vi "midiInOpen.vi"(7 "Event Filter":u8[](array[numeric])=[128, 144, 176] format="%.0x", 8 "error in":errorcluster, 9 "MidiDataEvents":refnum<user-event>, 10 "MIDI Device ID":u32, 11 "midi in":refnum<class "midi.lvclass">) -> (0 "error out":errorcluster, 3 "midi out":refnum<class "midi.lvclass">)   [LabVIEW 2020, in "midi.lvclass"]
doc: "The midiInOpen function opens a specified MIDI input device."
uses:
  midi.lvclass
  midi.lvclass/midi.ctl
  cpp-src/MIDIInToLabVIEWWrapper/x64/Release/MIDIInToLabVIEWWrapper.dll
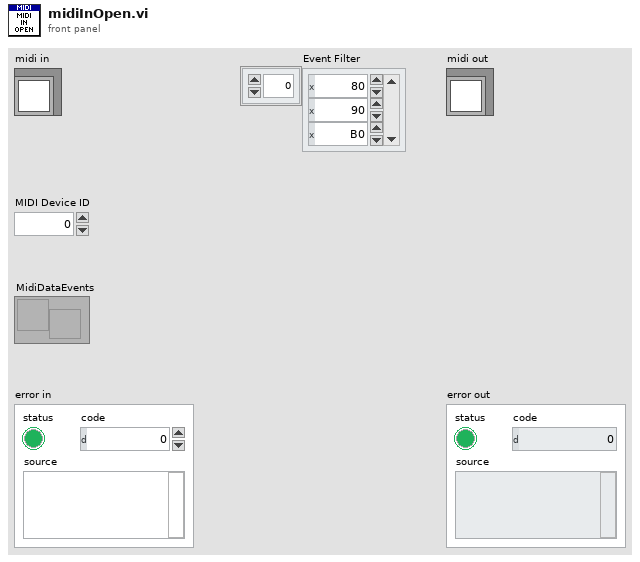
[diagram p1: front panel]
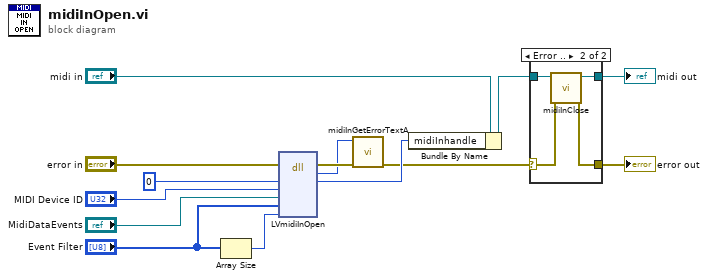
[diagram p0: block diagram]
diagram:
  n1 = Array Size(array="Event Filter") -> (size(s)=w2:i32)
  n2 = dll-call lib="C:/code/LabVIEW-MIDI/cpp-src/MIDIInToLabVIEWWrapper/x64/Release/MIDIInToLabVIEWWrapper.dll" fn="LVmidiInOpen"(error in="error in", "phMidiIn"=u64 0 ("hMidiIn"), "uDeviceID"="MIDI Device ID", "pUserEventRef"="MidiDataEvents", "filterArray"="Event Filter", "arraySize"=w2) -> (error out=w8:errorcluster, "error"=w7:i32, "phMidiIn"=w6:u64)  [unwired: 6 in, 1 out]
  n3 = call "midiInGetErrorTextA.vi"("error in"=w8, "Error Code"=w7) -> ("error out"=w5:errorcluster)  [unwired: 9 in]
  n4 = Bundle By Name(cluster="midi in", "midiInhandle"=w6) -> (w13:refnum<class "midi.lvclass">)
  n5 = case shown="Error .." w5 {
    selector: w5 -> [w15 w17]
    tunnel: w13 -> [w16 w20]
    tunnel: [w16 w19] -> w12
    tunnel: [w15 w18] -> w11
    frame No Error {
    }
    frame Error {
      n6 = call "midiInClose.vi"("error in"=w17, "midi in"=w20) -> ("error out"=w18:errorcluster, "midi out"=w19:refnum<class "midi.lvclass">)  [unwired: 8 in]
    }
  }
  "midi out" <- w12
  "error out" <- w11
